vi "sv_Edge Detection (No State).vi"(4 "state in":T1, 5 "reset? (True)":bool=TRUE, 6 "dt":dbl=11025.0, 8 "slope (Rising)":u16(ring) items=["Rising", "Falling"], 9 "pulse width (2)":i32=2, 10 "threshold (0.0)":dbl format="%.2f", 11 "x[n]":dbl[](array[numeric]) format="%.2f") -> (0 "state out":T1, 3 "pulse positions [s]":dbl[](array[numeric]) format="%.2f")   [LabVIEW 2012, in "Measurement Channels.lvlib" / "Tachometer.lvclass"]
doc: "Detects the edges in the tachometer pulses contained in <B>x[n]</B> that cross <B>threshold</B>. Perform edge detection to determine the tachometer pulse position. The VI recognizes the points where the signal crosses <B>threshold</B> and <B>x[n]</B> as edges. The VI returns the locations of the detected edges in <B>pulse positions [s]</B>."
uses:
  Tachometer.lvclass
  <vilib>/addons/Sound and Vibration/Order Analysis/Tach Process/SoundVib_TachProcess.lvlib
panel:
  # "Edge Detection (1 Tach)"
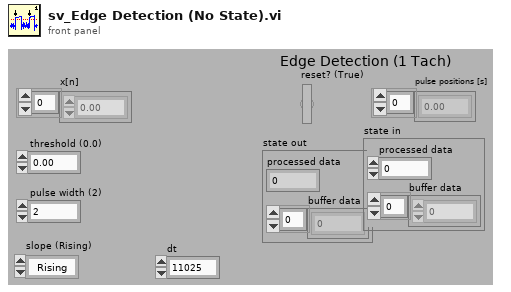
[diagram p1: front panel]
types:
  T1 = cluster{"processed data":dbl, "buffer data":dbl[]}
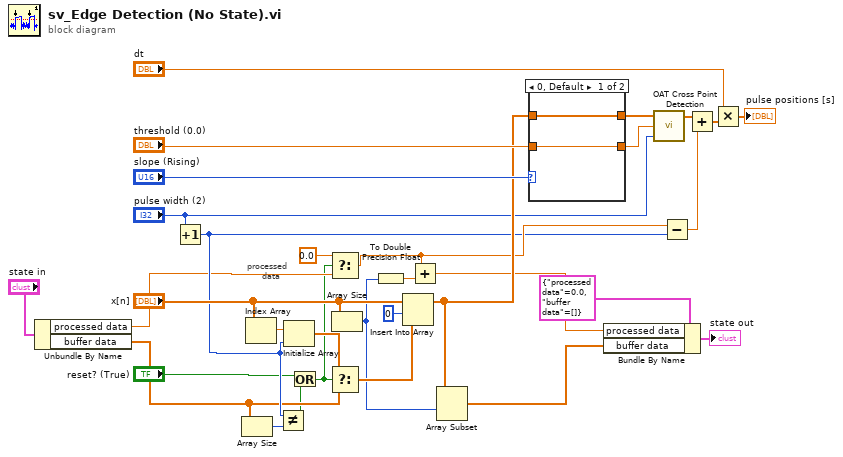
[diagram p0: block diagram]
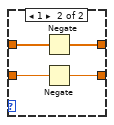
[diagram p2: hidden frame]
diagram:
  # "processed\n     data"
  n1 = Unbundle By Name("state in") -> ("processed data"=w13:dbl, "buffer data"=w12:dbl[])
  n2 = Increment(x="pulse width (2)") -> (x+1=w21:i32)
  n3 = Array Size(array=w12) -> (size(s)=w10:i32)
  n4 = Index Array(array="x[n]") -> (element=w11:dbl)  [unwired: 1 in]
  n5 = Not Equal?(x=w21, y=w10) -> (x != y?=w9:bool)
  n6 = Initialize Array(w11, w21) -> (w6:dbl[])
  n7 = Or(x="reset? (True)", y=w9) -> (x .or. y?=w5:bool)
  n8 = Select(t=0.0, s=w5, f=w13) -> (s? t:f=w24:dbl)
  n9 = Select(t=w6, s=w5, f=w12) -> (s? t:f=w8:dbl[])
  n10 = Array Size(array="x[n]") -> (size(s)=w3:i32)
  n11 = To Double Precision Float(number=w3) -> (double precision float=w2:dbl)
  n12 = Insert Into Array(array="x[n]", index=0 ("Index"), new element=w8) -> (w26:dbl[])
  n13 = Add(x=w24, y=w2) -> (x+y=w18:dbl)
  n14 = Array Subset(array=w26, index=w3) -> (w17:dbl[])  [unwired: 1 in]
  n15 = case shown="0, Default" "slope (Rising)" {
    tunnel: "threshold (0.0)" -> [w33 w36]
    tunnel: w26 -> [w34 w38]
    tunnel: [w34 w37] -> w29
    tunnel: [w33 w35] -> w31
    frame 0, Default {
    }
    frame 1 {
      n16 = Negate(x=w38) -> (-x=w37:dbl[])
      n17 = Negate(x=w36) -> (-x=w35:dbl)
    }
  }
  n18 = Bundle By Name(cluster=T1 {"processed data"=0.0, "buffer data"=[]}, "processed data"=w18, "buffer data"=w17) -> (→"state out":T1)
  n19 = call <vilib>:"OAT Cross Point Detection.vi"("pulse width (2)"="pulse width (2)", "threshold (0)"=w31, "data in"=w29) -> ("edge position"=w25:dbl[])  [unwired: 1 in]
  n20 = Subtract(x=w24, y=w21) -> (x-y=w22:dbl)
  n21 = Add(x=w25, y=w22) -> (x+y=w20:dbl[])
  n22 = Multiply(x="dt", y=w20) -> (x*y=→"pulse positions [s]":dbl[])
